vi "teleop ctrl pnl pi (SubVI).vi"() -> (3 "Numeric":dbl format="%#_50g")   [LabVIEW 2019]
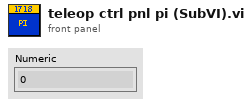
[diagram p1: front panel]
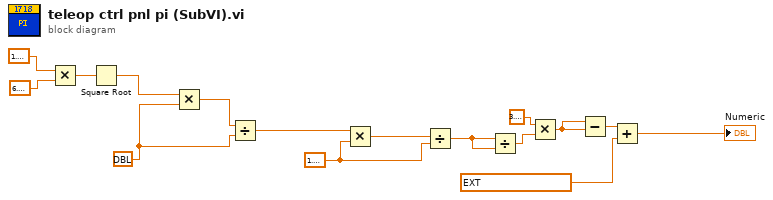
[diagram p0: block diagram]
diagram:
  w8 = 1.1447298858494002
  w13 = ext[unit] 6.0221408569999999998e+23
  n1 = Multiply(x=1.5707963267948966, y=6.283185307179586) -> (x*y=w11:dbl)
  n2 = Square Root(x=w11) -> (sqrt(x)=w10:dbl)
  n3 = Multiply(x=w10, y=w13) -> (x*y=w14:ext[unit])
  n4 = Divide(x=w14, y=w13) -> (x/y=w12:ext)
  n5 = Multiply(x=w12, y=w8) -> (x*y=w9:ext)
  n6 = Divide(x=w9, y=w8) -> (x/y=w7:ext)
  n7 = Divide(x=w7, y=w7) -> (x/y=w6:ext)
  n8 = Multiply(x=3.141592653589793, y=w6) -> (x*y=w4:ext)
  n9 = Subtract(x=w4, y=w4) -> (x-y=w3:ext)
  n10 = Add(x=w3, y=ext 3.14159265358979323) -> (x+y=→"Numeric":ext)
